vi "MeasurementServer_GetRequest_Config.vi"(6 "error in (no error)":errorcluster, 9 "gRPCid":T2) -> (0 "error out":errorcluster, 2 "ConfigRequest":T1, 3 "gRPCid out":T2)   [LabVIEW 2019, in "labview-grpc-measurement-server.lvlib"]
uses:
  labview-grpc-measurement-server.lvlib
  MeasurementServer_gRPCid.ctl
  MeasurementServer_ConfigRequest.ctl
  build/Debug/labview_measurement_server.dll
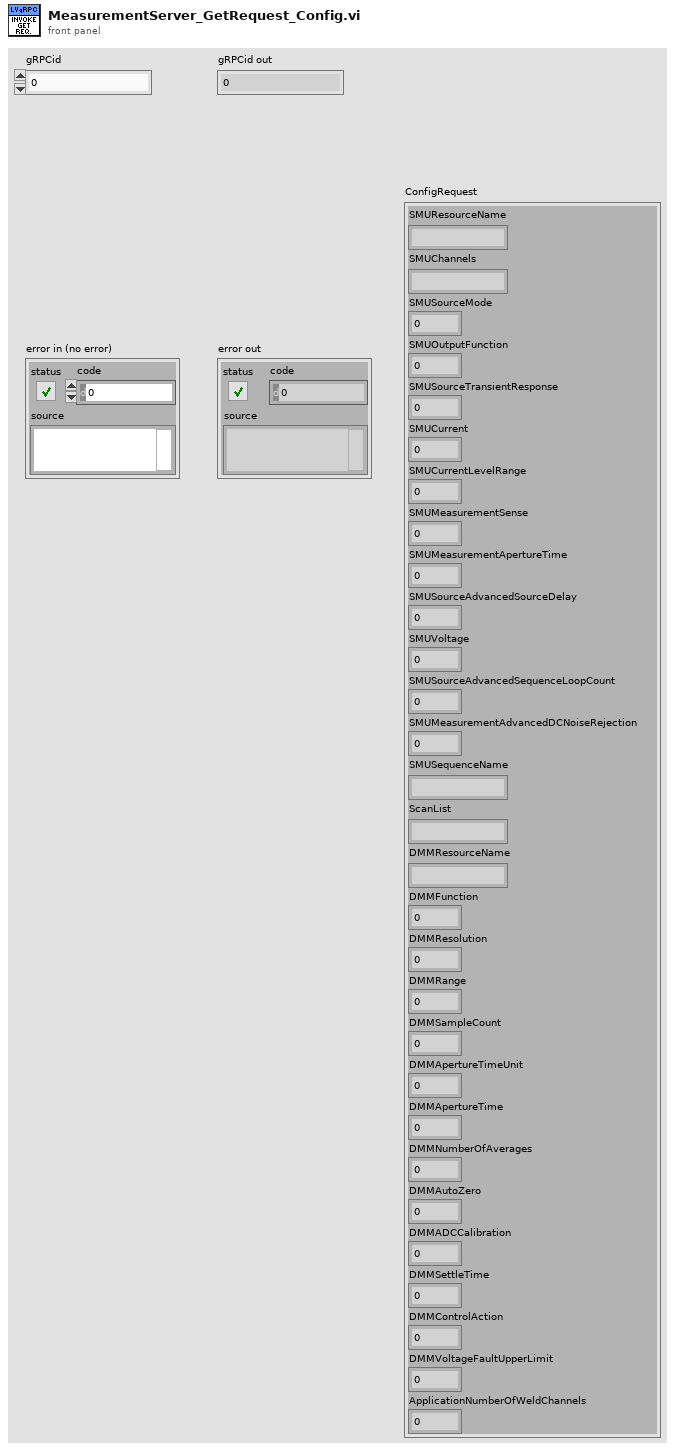
[diagram p1: front panel]
types:
  T1 = typedef "labview-grpc-measurement-server.lvlib/MeasurementServer_ConfigRequest.ctl" = cluster{"SMUResourceName":string, "SMUChannels":string, "SMUSourceMode":i32, "SMUOutputFunction":i32, "SMUSourceTransientResponse":i32, "SMUCurrent":sgl, "SMUCurrentLevelRange":sgl, "SMUMeasurementSense":i32, "SMUMeasurementApertureTime":sgl, "SMUSourceAdvancedSourceDelay":sgl, "SMUVoltage":sgl, "SMUSourceAdvancedSequenceLoopCount":i32, "SMUMeasurementAdvancedDCNoiseRejection":i32, "SMUSequenceName":string, "ScanList":string, "DMMResourceName":string, "DMMFunction":i32, "DMMResolution":sgl, "DMMRange":sgl, "DMMSampleCount":i32, "DMMApertureTimeUnit":i32, "DMMApertureTime":sgl, "DMMNumberOfAverages":i32, "DMMAutoZero":i32, "DMMADCCalibration":i32, "DMMSettleTime":sgl, "DMMControlAction":i32, "DMMVoltageFaultUpperLimit":sgl, "ApplicationNumberOfWeldChannels":i32}
  T2 = typedef "labview-grpc-measurement-server.lvlib/MeasurementServer_gRPCid.ctl" = u64
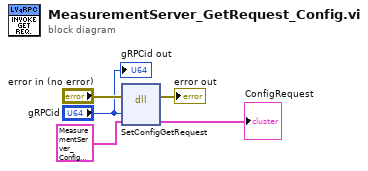
[diagram p0: block diagram]
diagram:
  n1 = dll-call lib="C:/dev/labview-grpc-measurement-server/build/Debug/labview_measurement_server.dll" fn="SetConfigGetRequest"(error in="error in (no error)", "id"="gRPCid", "data"=T1 {"SMUResourceName"="", "SMUChannels"="", "SMUSourceMode"=0, "SMUOutputFunction"=0, "SMUSourceTransientResponse"=0, "SMUCurrent"=0.0, "SMUCurrentLevelRange"=0.0, "SMUMeasurementSense"=0, "SMUMeasurementApertureTime"=0.0, "SMUSourceAdvancedSourceDelay"=0.0, "SMUVoltage"=0.0, "SMUSourceAdvancedSequenceLoopCount"=0, "SMUMeasurementAdvancedDCNoiseRejection"=0, "SMUSequenceName"="", "ScanList"="", "DMMResourceName"="", "DMMFunction"=0, "DMMResolution"=0.0, "DMMRange"=0.0, "DMMSampleCount"=0, "DMMApertureTimeUnit"=0, "DMMApertureTime"=0.0, "DMMNumberOfAverages"=0, "DMMAutoZero"=0, "DMMADCCalibration"=0, "DMMSettleTime"=0.0, "DMMControlAction"=0, "DMMVoltageFaultUpperLimit"=0.0, "ApplicationNumberOfWeldChannels"=0} ("ConfigRequest")) -> (error out=→"error out":errorcluster, "data"=→"ConfigRequest":T1)  [unwired: 4 in, 1 out]
  "gRPCid out" <- "gRPCid"
